vi "Remote Message.vi"(8 "Error In":errorcluster, 11 "Test LNA in":refnum<class "TestLNA.lvclass">) -> (0 "Error Out":errorcluster, 3 "Test LNA out":refnum<class "TestLNA.lvclass">)   [LabVIEW 2014, in "TestLNA.lvlib" / "TestLNA.lvclass"]
uses:
  TestLNA.lvclass
  CSPP_LNA/CS++LNAMessage.lvclass
  TestLNA.lvclass/TestLNA.ctl
  CSPP_LNA/CS++LNAMessage.lvclass/CS++LNAMessage.ctl
  CSPP_LNA/Write Message Class Name.vi
  CSPP_LNA/Write Parameter.vi
  <vilib>/NI/Actors/Linked Network Actor/Linked Network Actor Messages/Transmit Network Message Msg/Transmit Network Message Msg.lvclass
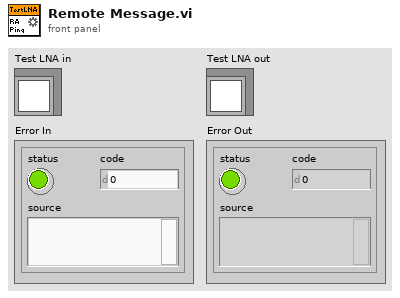
[diagram p1: front panel]
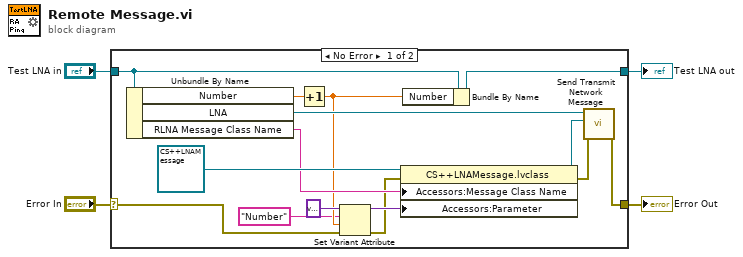
[diagram p0: block diagram]
diagram:
  n1 = case shown="No Error" "Error In" {
    selector: "Error In" -> [w6 w21]
    tunnel: [w18 w21] -> w3
    tunnel: [w12 w20] -> w1
    tunnel: "Test LNA in" -> [w13 w20]
    frame No Error {
      n2 = Unbundle By Name(w13) -> ("Number"=w11:dbl, "LNA"=w19:refnum<class "Message Enqueuer.lvclass">, "RLNA Message Class Name"=w16:string)
      n3 = Increment(x=w11) -> (x+1=w8:dbl)
      n4 = Set Variant Attribute(Variant=variant, name="Number", value=w8, error in=w6) -> (Variant out=w10:variant, error out=w5:errorcluster)  [unwired: 1 out]
      n5 = property class="CS++LNAMessage.lvclass"(reference=refnum<class "CS++LNAMessage.lvclass"> refnum ("CS++LNA.lvlib:CS++LNAMessage.lvclass"), error in=w5, "Accessors:Message Class Name"=w16, "Accessors:Parameter"=w10) -> (reference out=w14:refnum<class "CS++LNAMessage.lvclass">, error out=w15:errorcluster)
      n6 = Bundle By Name(cluster=w13, "Number"=w8) -> (w12:refnum<class "TestLNA.lvclass">)
      n7 = call <vilib>:"Send Transmit Network Message.vi"("error in (no error)"=w15, "Message"=w14, "Message Enqueuer"=w19) -> ("error out"=w18:errorcluster)  [unwired: 7 in, 1 out]
    }
    frame Error {
    }
  }
  "Error Out" <- w3
  "Test LNA out" <- w1
